vi "ExtractSpringDampers.vi"(4 "SpringDampers":T1(array[cluster])) -> (1 "SpringDampersDataOut":dbl[](array[numeric]))   [LabVIEW 2019]
panel:
  # "This VI accesses 10 springs or dampers saved within SpringDampers\n(10 because this is considered the max number used in our exercises)"
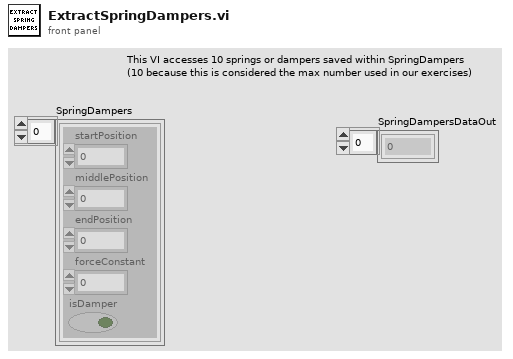
[diagram p1: front panel]
types:
  T1 = cluster{"startPosition":dbl, "middlePosition":dbl, "endPosition":dbl, "forceConstant":dbl, "isDamper":bool}[]
  T2 = cluster{"startPosition":dbl, "middlePosition":dbl, "endPosition":dbl, "forceConstant":dbl, "isDamper":bool}
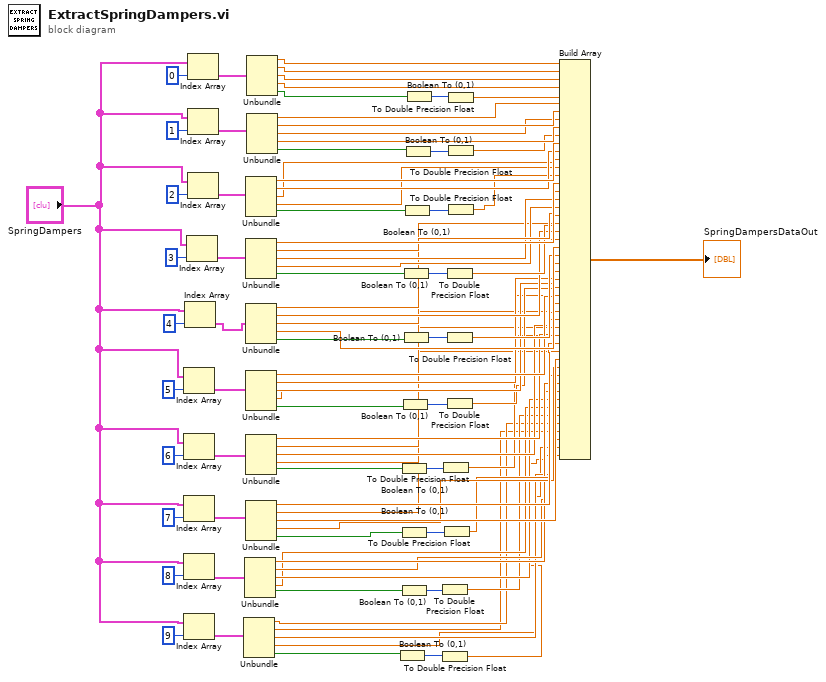
[diagram p0: block diagram]
diagram:
  n1 = Index Array(array="SpringDampers", index=5) -> (element=w76:T2)
  n2 = Index Array(array="SpringDampers", index=6) -> (element=w75:T2)
  n3 = Index Array(array="SpringDampers", index=7) -> (element=w74:T2)
  n4 = Index Array(array="SpringDampers", index=8) -> (element=w73:T2)
  n5 = Index Array(array="SpringDampers", index=9) -> (element=w72:T2)
  n6 = Index Array(array="SpringDampers", index=4) -> (element=w77:T2)
  n7 = Index Array(array="SpringDampers", index=3) -> (element=w78:T2)
  n8 = Index Array(array="SpringDampers", index=0) -> (element=w91:T2)
  n9 = Index Array(array="SpringDampers", index=1) -> (element=w80:T2)
  n10 = Index Array(array="SpringDampers", index=2) -> (element=w79:T2)
  n11 = Unbundle(w72) -> ("startPosition"=w7:dbl, "middlePosition"=w6:dbl, "endPosition"=w5:dbl, "forceConstant"=w4:dbl, "isDamper"=w3:bool)
  n12 = Unbundle(w73) -> ("startPosition"=w13:dbl, "middlePosition"=w12:dbl, "endPosition"=w11:dbl, "forceConstant"=w10:dbl, "isDamper"=w8:bool)
  n13 = Unbundle(w79) -> ("startPosition"=w61:dbl, "middlePosition"=w60:dbl, "endPosition"=w59:dbl, "forceConstant"=w58:dbl, "isDamper"=w57:bool)
  n14 = Unbundle(w78) -> ("startPosition"=w56:dbl, "middlePosition"=w42:dbl, "endPosition"=w41:dbl, "forceConstant"=w40:dbl, "isDamper"=w38:bool)
  n15 = Unbundle(w77) -> ("startPosition"=w37:dbl, "middlePosition"=w36:dbl, "endPosition"=w35:dbl, "forceConstant"=w34:dbl, "isDamper"=w33:bool)
  n16 = Unbundle(w76) -> ("startPosition"=w31:dbl, "middlePosition"=w30:dbl, "endPosition"=w29:dbl, "forceConstant"=w28:dbl, "isDamper"=w27:bool)
  n17 = Unbundle(w75) -> ("startPosition"=w25:dbl, "middlePosition"=w24:dbl, "endPosition"=w23:dbl, "forceConstant"=w22:dbl, "isDamper"=w20:bool)
  n18 = Unbundle(w74) -> ("startPosition"=w19:dbl, "middlePosition"=w18:dbl, "endPosition"=w17:dbl, "forceConstant"=w16:dbl, "isDamper"=w15:bool)
  n19 = Unbundle(w91) -> ("startPosition"=w71:dbl, "middlePosition"=w70:dbl, "endPosition"=w69:dbl, "forceConstant"=w68:dbl, "isDamper"=w67:bool)
  n20 = Unbundle(w80) -> ("startPosition"=w66:dbl, "middlePosition"=w65:dbl, "endPosition"=w64:dbl, "forceConstant"=w63:dbl, "isDamper"=w62:bool)
  n21 = Boolean To (0,1)(Boolean=w3) -> (0, 1=w45:i16)
  n22 = Boolean To (0,1)(Boolean=w20) -> (0, 1=w48:i16)
  n23 = Boolean To (0,1)(Boolean=w15) -> (0, 1=w47:i16)
  n24 = Boolean To (0,1)(Boolean=w8) -> (0, 1=w46:i16)
  n25 = Boolean To (0,1)(Boolean=w27) -> (0, 1=w49:i16)
  n26 = Boolean To (0,1)(Boolean=w38) -> (0, 1=w51:i16)
  n27 = Boolean To (0,1)(Boolean=w33) -> (0, 1=w50:i16)
  n28 = Boolean To (0,1)(Boolean=w57) -> (0, 1=w52:i16)
  n29 = Boolean To (0,1)(Boolean=w62) -> (0, 1=w53:i16)
  n30 = Boolean To (0,1)(Boolean=w67) -> (0, 1=w55:i16)
  n31 = To Double Precision Float(number=w46) -> (double precision float=w9:dbl)
  n32 = To Double Precision Float(number=w45) -> (double precision float=w2:dbl)
  n33 = To Double Precision Float(number=w48) -> (double precision float=w21:dbl)
  n34 = To Double Precision Float(number=w47) -> (double precision float=w14:dbl)
  n35 = To Double Precision Float(number=w51) -> (double precision float=w39:dbl)
  n36 = To Double Precision Float(number=w50) -> (double precision float=w32:dbl)
  n37 = To Double Precision Float(number=w49) -> (double precision float=w26:dbl)
  n38 = To Double Precision Float(number=w55) -> (double precision float=w54:dbl)
  n39 = To Double Precision Float(number=w53) -> (double precision float=w44:dbl)
  n40 = To Double Precision Float(number=w52) -> (double precision float=w43:dbl)
  n41 = Build Array(w71, w70, w69, w68, w54, w66, w65, w64, w63, w44, w61, w60, w59, w58, w43, w56, w42, w41, w40, w39, w37, w36, w35, w34, w32, w31, w30, w29, w28, w26, w25, w24, w23, w22, w21, w19, w18, w17, w16, w14, w13, w12, w11, w10, w9, w7, w6, w5, w4, w2) -> (→"SpringDampersDataOut":dbl[])
